vi "Magnet Global.vi"() -> ()   [LabVIEW 2009, in "Magnet.lvclass"]
uses:
  Magnet.lvclass
panel:
  out "Stop":bool
  out "Interrupt":bool
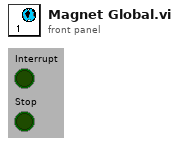
[diagram p1: front panel]
diagram:
